vi "create Board.vi"(4 "Height":i32, 6 "Width":i32, 8 "error in (no error)":errorcluster, 10 "Players":refnum<class "Player.lvclass">[](array[class]), 11 "Board in":refnum<class "Board.lvclass">) -> (0 "error out":errorcluster, 3 "Board out":refnum<class "Board.lvclass">)   [LabVIEW 2019, in "Board.lvclass"]
uses:
  Board.lvclass
  Player/Player.lvclass
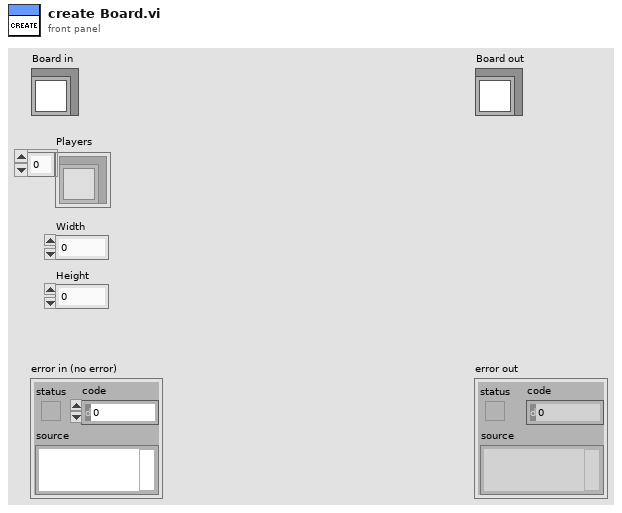
[diagram p1: front panel]
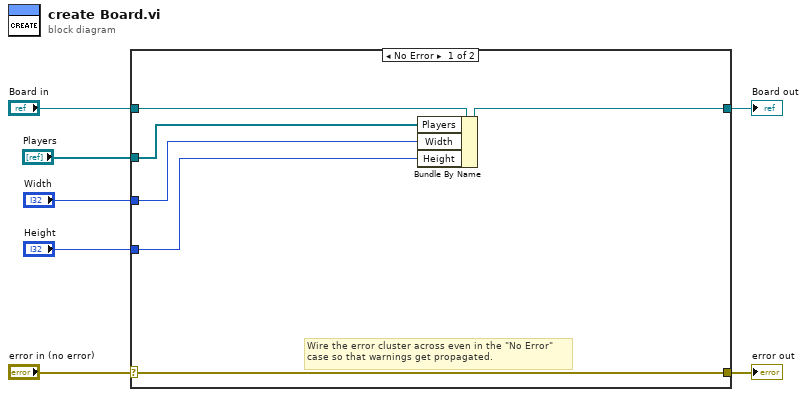
[diagram p0: block diagram]
diagram:
  n1 = case shown="No Error" "error in (no error)" {
    selector: "error in (no error)" -> [w12 w15]
    tunnel: [w12 w15] -> w6
    tunnel: [w11 w14] -> w4
    tunnel: "Board in" -> [w13 w14]
    tunnel: "Players" -> [w10 _]
    tunnel: "Width" -> [w9 _]
    tunnel: "Height" -> [w8 _]
    frame No Error {
      # "Wire the error cluster across even in the \"No Error\"\ncase so that warnings get propagated."
      n2 = Bundle By Name(cluster=w13, "Players"=w10, "Width"=w9, "Height"=w8) -> (w11:refnum<class "Board.lvclass">)
    }
    frame Error {
    }
  }
  "error out" <- w6
  "Board out" <- w4
